vi "读取配置信息 (子VI).vi"(8 "error in (no error)":errorcluster caption="错误输入（无错误）") -> (0 "错误输出":errorcluster)   [LabVIEW 2022 SP3, in "超标留样集成.lvlib"]
uses:
  <vilib>/Utility/config.llb/NI_LVConfig.lvlib
  <userlib>/_OpenG.lib/variantconfig/variantconfig.llb/openg_variant_configuration_file.lvlib
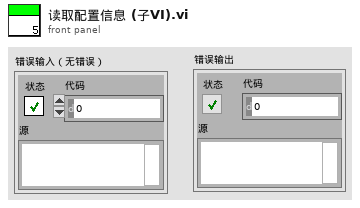
[diagram p1: front panel]
types:
  T1 = typedef "NI_LVConfig.lvlib/Config Data RefNum.ctl" = refnum<k1>
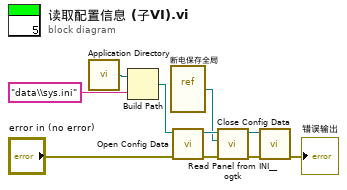
[diagram p0: block diagram]
diagram:
  n1 = call <vilib>:"Application Directory.vi"() -> ("Application Directory"=w9:path)
  n2 = Build Path(base path=w9, name or relative path="data\\sys.ini" ("名称或相对路径")) -> (appended path=w7:path)
  n3 = vi-ref "断电保存全局.vi"() -> (w5:refnum<vi>)
  n4 = call <vilib>:"Open Config Data.vi"("error in (no error)"="error in (no error)", "configuration file path"=w7) -> ("error out"=w3:errorcluster, "refnum"=w6:T1)  [unwired: 7 in, 1 out]
  n5 = call <userlib>:"Read Panel from INI__ogtk.vi"("error in (no error)"=w3, "VI ref"=w5, "refnum"=w6) -> ("error out"=w2:errorcluster, "refnum out"=w4:T1)  [unwired: 7 in]
  n6 = call <vilib>:"Close Config Data.vi"("error in (no error)"=w2, "refnum"=w4) -> ("error out"=→"错误输出":errorcluster)  [unwired: 8 in, 1 out]
